vi "stop.vi"(8 "error in (no error)":errorcluster, 9 "CameraSettings":refnum<class "CamaraSettings.lvclass">, 10 "stop":bool, 11 "ProEM_WinX32 in":refnum<class "ProEM_WinX32.lvclass">) -> (0 "error out":errorcluster, 1 "imageSaved":bool, 2 "stopped?":bool, 3 "ProEM_WinX32 out":refnum<class "ProEM_WinX32.lvclass">)   [LabVIEW 2009, in "Hardware.lvlib" / "Channels.lvlib" / "ProEM_WinX32.lvclass"]
uses:
  ProEM_WinX32.lvclass
  Tools/CameraSettings/CamaraSettings.lvclass
  ProEM_WinX32.lvclass/ProEM_WinX32.ctl
  Camera/Camera.lvclass
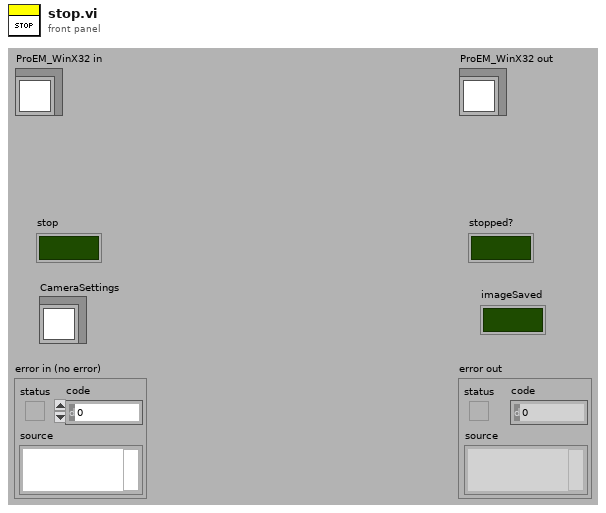
[diagram p1: front panel]
types:
  T1 = typedef "WINX32 Object Reference.ctl" = refnum<k1>
  T2 = typedef "WINX32 Data Members.ctl" = cluster{"WINX32Lib.IExpSetup":refnum<k7>, "WINX32Lib.IDocFile":refnum<k7>, "Result Image":T3, "Image to save":T3, "hardware present":bool, "started?":bool, "Image array from WINX":u16[][][], "raw images":cluster{"2D Image Array":u16[][]}[], "Camera active":bool, "images":T4, "Camera":T5}
  T3 = typedef "IMAQ Image.ctl" = refnum<image>
  T4 = typedef "WINX32 Image.ctl" = cluster{"processed":cluster{"Image":T3, u32}, "object":cluster{"Image":T3, u32}, "background":cluster{"Image":T3, u32}, "reference":cluster{"Image":T3, u32}, "mask":cluster{"Image":T3, u32}, "ROI Descriptor":cluster{"Global Rectangle":i32[], "Contours":cluster{"ID":enum32{"External", "Internal"}, "Type":enum32{"No Selection", "Point", "Line", "Rectangle", "Oval", "Polygon", "Free", "Unused1", "Unused2", "Unused3", "Broken Line", "Free Hand Line"}, "Coordinates":i32[]}[]}}
  T5 = typedef "Analyse - Camera.ctl" = cluster{"Bit Range(1023)":u32, "step(1.88)":dbl}
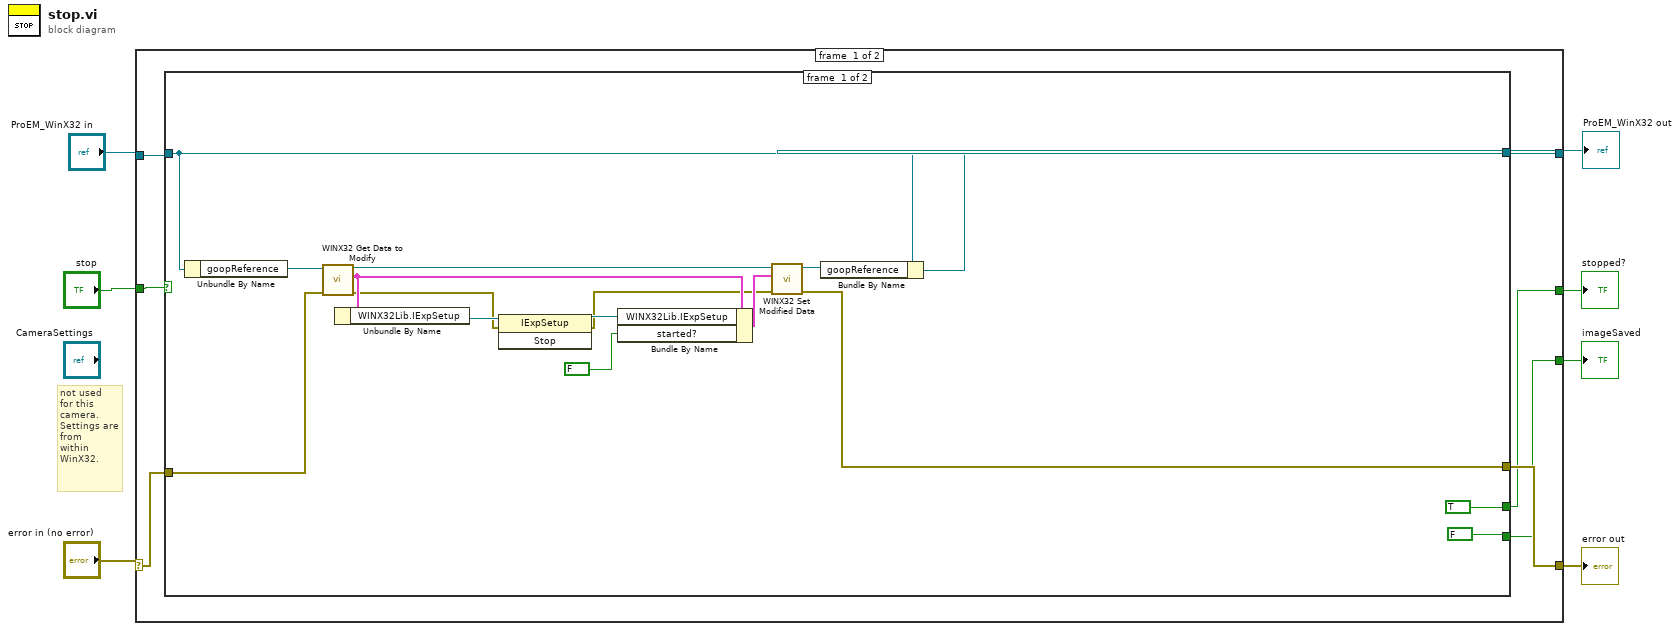
[diagram p0: block diagram]
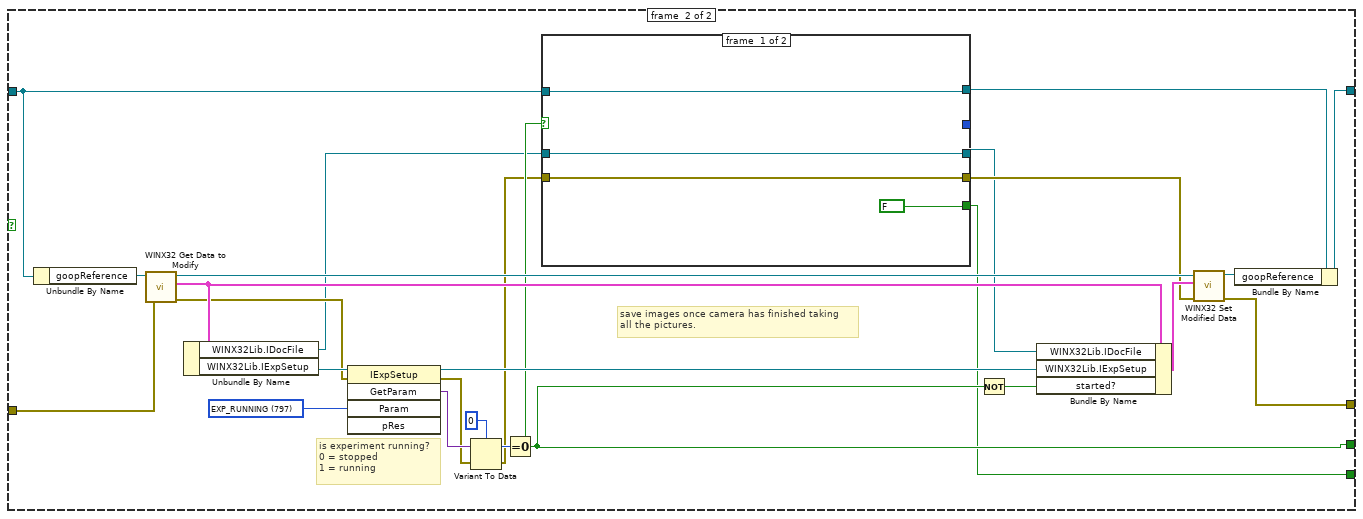
[diagram p2: hidden frame]
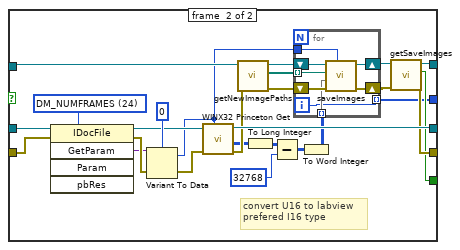
[diagram p3: hidden frame]
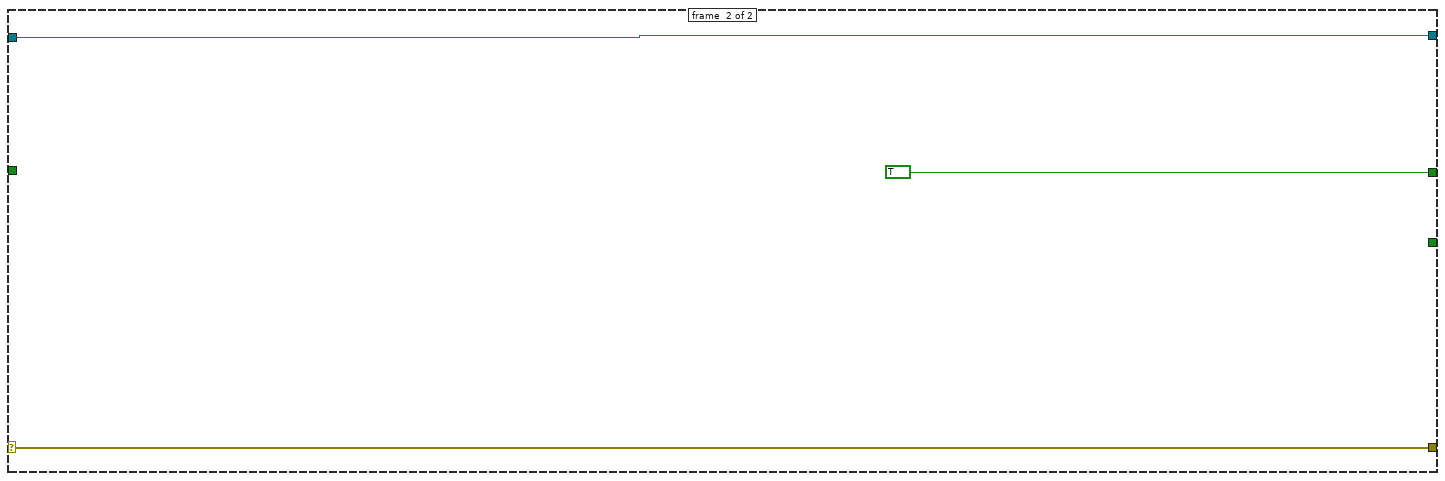
[diagram p4: hidden frame]
diagram:
  # "not used \nfor this\ncamera.\nSettings are\nfrom \nwithin \nWinX32."
  n1 = case shown="No Error" "error in (no error)" {
    selector: "error in (no error)" -> [w14 w95]
    tunnel: [w11 w96] -> w6
    tunnel: "ProEM_WinX32 in" -> [w12 w96]
    tunnel: [w10 w95] -> w4
    tunnel: "stop" -> [w13 _]
    tunnel: [w9 TRUE] -> w2
    tunnel: [w8 _] -> w1
    frame #0 {
      n2 = case shown="False" w13 {
        tunnel: w12 -> [w30 w32]
        tunnel: w14 -> [w27 w53]
        tunnel: [w29 w55] -> w11
        tunnel: [w17 w46] -> w10
        tunnel: [TRUE w38] -> w9
        tunnel: [FALSE w31] -> w8
        frame #0 {
          n3 = Unbundle By Name(w30) -> ("goopReference"=w28:T1)
          n4 = call <instrlib>:"WINX32 Get Data to Modify.vi"("error in (no error)"=w27, "reference"=w28) -> ("error out"=w23:errorcluster, "data"=w25:T2, "duplicate reference"=w21:T1)  [unwired: 2 in, 1 out]
          n5 = Unbundle By Name(w25) -> ("WINX32Lib.IExpSetup"=w26:refnum<k7>)
          n6 = invoke class="IExpSetup" method="Stop"(reference=w26, error in=w23) -> (reference out=w24:refnum<k7>, error out=w19:errorcluster)  [unwired: 1 in, 1 out]
          n7 = Bundle By Name(cluster=w25, "WINX32Lib.IExpSetup"=w24, "started?"=FALSE) -> (w20:T2)
          n8 = call <instrlib>:"WINX32 Set Modified Data.vi"("error in (no error)"=w19, "data"=w20, "reference"=w21) -> ("error out"=w17:errorcluster, "duplicate reference"=w22:T1)  [unwired: 3 in]
          n9 = Bundle By Name(cluster=w30, "goopReference"=w22) -> (w29:refnum<class "ProEM_WinX32.lvclass">)
        }
        frame #1 {
          w45 = 797 items=["EXP_ETACTUAL"=1, "EXP_SEQUENTS"=2, "EXP_ERROR"=3, "EXP_GETCAPS"=4, "EXP_GETPLSR"=5, "EXP_DETECTOR_BIT"=16, "EXP_RUNNING_APP"=23, "EXP_VIDEO_TYPE"=24, "EXP_CUSTOM_VIDEO_X"=25, "EXP_CUSTOM_VIDEO_Y"=26, "EXP_CUSTOM_VIDEO_FSTWIDTH"=27, "EXP_CUSTOM_VIDEO_LSTWIDTH"=28, "EXP_VIDEO_XDIM"=29, "EXP_VIDEO_YDIM"=30, "EXP_VIDEO_MAX_ZOOM"=31, "EXP_VIDEO_HORZ_PAN"=32, "EXP_VIDEO_VERT_PAN"=33, "EXP_WORD_MULTIPLIER"=34, "EXP_TARGET_ID"=35, "EXP_ADAPTER_ID"=36, "EXP_NUMADAPTORS"=37, "EXP_FORCE_PP_INIT"=38, "EXP_NOP_ADC"=39, "EXP_ACTUAL_TEMP"=40, "EXP_FORCE_AUTOSTOP"=41, "EXP_DEFAULT_VTCLK"=42, "EXP_MIN_VTCLK"=43, "EXP_MAX_VTCLK"=44, "EXP_DEFAULT_HTCLK"=45, "EXP_MIN_HTCLK"=46, "EXP_MAX_HTCLK"=47, "EXP_TIMING_STYLE"=48, "EXP_HEADSELECT"=49, "EXP_HORZPHASE"=50, "EXP_VERTPHASE"=51, "EXP_SPECIAL_SPEED"=52, "EXP_PRE_STRIPS"=53, "EXP_POST_STRIPS"=54, "EXP_PRE_LINES"=55, "EXP_POST_LINES"=56, "EXP_ACTIVE_LINES"=57, "EXP_ACTIVE_STRIPS"=58, "EXP_XFER_EXTRA"=59, "EXP_MIN_BLOCK"=60, "EXP_NUM_MIN_BLOCK"=61, "EXP_LOGIC_OUTPUT"=66, "EXP_VIDEO_BLANK"=67, "EXP_ZOOM_MODE_VIDEO"=68, "EXP_LEVEL_SYNC"=69, "EXP_DISABLE_LASER"=70, "EXP_ACQBACK_SHUTTER"=71, "EXP_ACQFLAT_SHUTTER"=72, "EXP_SMALL_CCD_MINEXP"=73, "EXP_LARGE_CCD_MINEXP"=74, "EXP_GATING_MODE"=75, "EXP_ILME_B1X"=76, "EXP_ILME_B2X"=77, "EXP_ILME_D1X"=78, "EXP_ILME_D2X"=79, "EXP_ILME_D4X"=80, "EXP_INIT_HW_ACCUM"=81, "EXP_5X_GAIN_ENABLE"=82, "EXP_RET_SRCCMP"=83, "EXP_EVENT_HANDLE"=84, "EXP_READOUT_MODE"=85, "EXP_SHUTTER_TYPE"=86, "EXP_USER_DEFINED_CHIP"=87, "EXP_USER_DEFINED_TIMING"=88, "EXP_CONTROLLER_VERSION"=89, "EXP_GET_CONTROLLER_VER"=90, "EXP_TTL_LINES"=91, "EXP_BIT_ADJUST"=92, "EXP_RESOLUTION"=93, "EXP_GAIN"=94, "EXP_ADC_RATE"=95, "EXP_ADC_TYPE"=96, "EXP_NUMBER_OF_CLEANS"=97, "EXP_NUM_OF_STRIPS_PER_CLN"=98, "EXP_INTERFACE_CARD"=99, "EXP_INTERRUPT"=100, "EXP_IO_ADDRESS1"=101, "EXP_IO_ADDRESS2"=102, "EXP_IO_ADDRESS3"=103, "EXP_HW_ROI"=104, "EXP_HW_BINNING"=105, "EXP_EDGE_TRIGGER"=106, "EXP_SHUTTER_CONTROL"=107, "EXP_RS170"=108, "EXP_RS170_COMPLEX"=109, "EXP_HW_RS170_LUT"=110, "EXP_RS170_INTENSITY_SCALING"=111, "EXP_RS170_OFFSET"=112, "EXP_RS170_PAN"=113, "EXP_RS170_ZOOM2X"=114, "EXP_RS170_ZOOM4X"=115, "EXP_RS170_BINNING"=116, "EXP_RS170_DECIMATION"=117, "EXP_HW_ACCUM"=118, "EXP_SHT_PREOPEN"=119, "EXP_STORE_STROBE"=120, "EXP_CONT_CLNS"=121, "EXP_TIMING_MODE"=122, "EXP_EXT_TRIGGER"=123, "EXP_EVENT_COUNTER"=124, "EXP_SW_TRIGGER"=125, "EXP_KINETICS_WINDOWSIZE"=126, "EXP_EXPOSURE"=127, "EXP_CONTROLLER_NAME"=128, "EXP_CCD_CHIP_NAME"=129, "EXP_BSWBINNING"=297, "EXP_EDGEENHANCE"=130, "EXP_BOXVIDEOGAIN"=131, "EXP_HSHADING_VALUE"=132, "EXP_VSHADING_VALUE"=133, "EXP_EDGEENHANCE_FLAG"=134, "EXP_SHADING_FLAG"=135, "EXP_GRAYSCALE"=136, "EXP_OFFSET"=137, "EXP_CCDGAIN"=138, "EXP_TEMPERATURE"=139, "EXP_MCPVOLTAGE"=140, "EXP_BOXEXPOSURE"=141, "EXP_ABC_FLAG"=142, "EXP_GAMMA_FLAG"=143, "EXP_AUTOBLACK_FLAG"=144, "EXP_AGC_FLAG"=145, "EXP_ODD_FIELD"=146, "EXP_FIELD_SELECT"=147, "EXP_RESET"=148, "EXP_EXTERN_ENABLE"=149, "EXP_CONTROLLERS_SUPPORTED"=150, "EXP_VTCLK"=151, "EXP_HTCLK"=152, "EXP_GATE_VS_CW"=153, "EXP_COM_PORT"=154, "EXP_US_UNITS"=156, "EXP_MS_UNITS"=157, "EXP_SEC_UNITS"=158, "EXP_MIN_UNITS"=159, "EXP_HRS_UNITS"=160, "EXP_FRAME_UNITS"=161, "EXP_SYNC_ASYNC"=162, "EXP_FOCUS_NFRAME"=163, "EXP_TIMEOUT"=164, "EXP_TIMEOUT_DEFAULT"=165, "EXP_HW_AUTOSTOP"=166, "EXP_RS170_INTEN_OFFSET"=167, "EXP_CONTROLLER_ALIVE"=168, "EXP_FOCUS_TYPE"=169, "EXP_FOCUS_ZOOM"=170, "EXP_FOCUS_PAN"=171, "EXP_MULTI_TAP_ROI"=172, "EXP_USE_INTERUPTS"=173, "EXP_DATA_ACQ_STATE"=174, "EXP_VERIFY_GOOD_VALUES"=175, "EXP_WHITE_CLAMP"=176, "EXP_BLACK_CLAMP"=177, "EXP_DELAY_TIME"=178, "EXP_READOUT_TIME"=179, "EXP_SW_DIAG"=180, "EXP_DIAG1"=181, "EXP_DIAG2"=182, "EXP_DIAG3"=183, "EXP_DIAG4"=184, "EXP_DIAG5"=185, "EXP_AorB_GROUP"=186, "EXP_ABSORBANCE_FLAG"=187, "EXP_ABSORBANCE_METHOD"=188, "EXP_ABSORBANCE_STRIPNUM"=189, "EXP_DMASIZE_VIA_DRIVER"=190, "EXP_DRIVERVERSION"=191, "EXP_NUM_DEVICES"=192, "EXP_ECPDMA_CHANNEL"=193, "EXP_CUSTOM_SHUTTER"=194, "EXP_ADC_OFFSET"=195, "EXP_CURRENT_READOUT_MODE"=196, "EXP_BANK_ADD"=197, "EXP_LUT_BANK"=198, "EXP_SETUP_STATUS"=201, "EXP_XY_GROUPING"=239, "EXP_MESSAGES_FLAG"=240, "EXP_TTL_LINE_TO_WAIT"=253, "EXP_DATA_COLLECTION_MODE"=258, "EXP_DATA_COLLECTION_TYPE"=262, "EXP_SKIPFRAMES"=274, "EXP_CLR_INT_CNTR"=276, "EXP_ENABLE_INT_CNTR"=277, "EXP_INT_CNTR"=278, "EXP_INTERNAL_SYNC_SRC"=279, "EXP_SW_EXTSYNC"=280, "EXP_PTG_PRESENT"=281, "EXP_ELEC_SHT"=282, "EXP_BOARDS_WITH_NVRAM"=283, "EXP_ANLGMASTER_ST143"=284, "EXP_ANLGSLAVE_ST143"=285, "EXP_DISPLAY_ST143"=286, "EXP_INTRFACE_ST143"=287, "EXP_SCANCONTROL_ST143"=288, "EXP_NUMBERFRAMES_IRQ"=204, "EXP_COOL_TYPE"=214, "EXP_HD_TYPE"=215, "EXP_INTENSIFER_GAIN"=216, "EXP_SHT_GATE_MODE"=217, "EXP_HD_CHECK"=218, "EXP_AMP_MODE"=219, "EXP_AMP_DIALOG"=247, "EXP_ANALOG_GAIN"=220, "EXP_HW_FIXES"=221, "EXP_PCI_CARDS"=222, "EXP_NOT_REVERSE"=223, "EXP_LOAD_NVRAM_DEFAULTS"=234, "EXP_CNTR_BRD"=235, "EXP_XDIMHW"=237, "EXP_YDIMHW"=238, "EXP_SPECIAL_FAST_RDOUT"=254, "EXP_SPCL_FAST_Y_DIM"=255, "EXP_SPCL_FAST_X_DIM"=256, "EXP_SPCL_FAST_Y_INDEX"=257, "EXP_SHUTTER_COMP_TIME_MS"=266, "EXP_NVRAM_AVAIL"=267, "EXP_NUMBER_AGAIN_AVAIL"=269, "EXP_SENSOR_TYPE"=270, "EXP_EVENT_TYPE"=292, "EXP_ANTI_BLOOMING"=293, "EXP_FAST_PULSE_ENABLE"=233, "EXP_USE_HEADCALIB"=296, "EXP_TEMP_STATUS"=301, "EXP_MULTIPLE_READMODES_LIVE"=302, "EXP_FIRST_ACQUIRE_FLAG"=303, "EXP_ANTI_BLOOMING_CONTROL"=304, "EXP_PRE_HORZ_DELAY"=305, "EXP_NVRAM_TRIES"=306, "EXP_XASCEND"=307, "EXP_YASCEND"=308, "EXP_ALT_TIMING"=309, "EXP_SHUTTER_PRE_COMP"=310, "EXP_PVCAM_POSSIBLE"=311, "EXP_ADC_IN_NVRAM"=312, "EXP_PASSTHRU_MODE"=313, "EXP_FIRMWAREVERSION"=314, "EXP_IMMEDIATE_SHUTTER"=315, "EXP_STAGE2_TEMP"=316, "EXP_AVGAIN_ENABLED"=317, "EXP_AVGAIN_SETPOINT"=318, "EXP_AVGAIN"=319, "EXP_AVGAIN_CALIB_TEMP"=320, "EXP_AVGAIN_CALIB_COEFF1"=321, "EXP_AVGAIN_CALIB_COEFF2"=322, "EXP_AVGAIN_CALIB_COEFF3"=323, "EXP_AVGAIN_CALIB_COEFF4"=324, "EXP_AVGAIN_CALIB_COEFF5"=325, "EXP_FORCE_READOUT_MODE"=326, "EXP_RESET_DATACOLLECTION"=327, "EXP_ACTIVE_SUBFRAME"=328, "EXP_PV_READOUT_PORT"=514, "EXP_CLASSNAME"=775, "EXP_FLATFLDNAME"=776, "EXP_DARKNAME"=777, "EXP_SETUPNAME"=778, "EXP_ACCESSNAME"=779, "EXP_DATFILENAME"=780, "EXP_ABSORBFILENAME"=781, "EXP_BLEMISHFILENAME"=782, "EXP_COSMICFILENAME"=783, "EXP_FILEINCBASENAME"=784, "EXP_YTNAME"=785, "EXP_DEVNAME"=786, "EXP_USEROI"=787, "EXP_DOBLEMISH"=788, "EXP_DOABSORB"=789, "EXP_DOCOSMIC"=790, "EXP_COSMICSENS"=791, "EXP_ABSORBSTRIP"=792, "EXP_DATATYPE"=793, "EXP_OVERWRITECONFIRM"=794, "EXP_FILEINCENABLE"=795, "EXP_FILEINCCOUNT"=796, "EXP_RUNNING"=797, "EXP_SAVEROPT"=798, "EXP_TIME_UNITS"=799, "EXP_FILEACCESS"=800, "EXP_AUTOSAVE"=801, "EXP_NEWWINDOW"=802, "EXP_XDIM"=803, "EXP_YDIM"=804, "EXP_XDIMDET"=805, "EXP_YDIMDET"=806, "EXP_ROIMODE"=807, "EXP_NUMREPEATSEXP"=808, "EXP_NUMACCUMSEXP"=809, "EXP_THREADSTATE"=810, "EXP_USEMINTHRESHOLDING"=811, "EXP_MINTHRESHOLDVALUE"=812, "EXP_USEMAXTHRESHOLDING"=813, "EXP_MAXTHRESHOLDVALUE"=814, "EXP_RUNNING_EXPERIMENT"=815, "EXP_THRESHOLD_DEMAND_UPDATE"=816, "EXP_ROICOUNT"=817, "EXP_ACCUMS"=818, "EXP_CACCUMS"=819, "EXP_CSEQUENTS"=820, "EXP_PHOTON_ESTIMATION_ENABLE"=821, "EXP_PHOTON_MAXTIME"=822, "EXP_PHOTON_MAXTIMEUNIT"=823, "EXP_CUSTOMFILTER_ENABLE"=824, "EXP_CUSTOMFILTER_SIZE"=825, "EXP_LOOKUPTABLE_ENABLE"=826, "EXP_BSHOWWINDOW"=827, "EXP_BBACKSUBTRACT"=828, "EXP_BDOFLATFIELD"=829, "EXP_ASCIIOUTPUTFILE"=830, "EXP_ASCIIOUTPUT_DELIMITER"=831, "EXP_ASCIIOUTPUT_TERMINATOR"=832, "EXP_FFTYPE"=833, "EXP_BGTYPE"=834, "EXP_COSGRASS"=835, "EXP_RUNASCONFIRM"=836, "EXP_RUNASRUNACCESS"=837, "EXP_DATAFILETYPE"=838, "EXP_ROTATE"=839, "EXP_FLIP"=840, "EXP_REVERSE"=841, "EXP_SWBINNING"=842, "EXP_AUTOSTORE"=843, "EXP_XBINNED"=844, "EXP_YBINNED"=845, "EXP_NUMPATTERNS"=846, "EXP_EXPERIMENTTIME"=847, "EXP_ASYNCSEQUENTIALS"=848, "EXP_SEQUENTIALS"=849, "EXP_CSEQUENTIALS"=850, "EXP_AUTOD"=851, "EXP_EXPOSURETIME"=852, "EXP_EXPOSURETIME_UNITS"=853, "EXP_ACQMODE"=854, "EXP_DMASIZE_PVCAM"=855, "EXP_INITIALIZE"=856, "EXP_CELL_X_SIZE"=857, "EXP_CELL_Y_SIZE"=858, "EXP_X_GAP_SIZE"=859, "EXP_Y_GAP_SIZE"=860] ("Param")
          # "is experiment running?\n0 = stopped\n1 = running"
          # "save images once camera has finished taking\nall the pictures."
          n10 = Unbundle By Name(w32) -> ("goopReference"=w54:T1)
          n11 = call <instrlib>:"WINX32 Get Data to Modify.vi"("error in (no error)"=w53, "reference"=w54) -> ("error out"=w50:errorcluster, "data"=w51:T2, "duplicate reference"=w48:T1)  [unwired: 2 in, 1 out]
          n12 = Unbundle By Name(w51) -> ("WINX32Lib.IDocFile"=w35:refnum<k7>, "WINX32Lib.IExpSetup"=w52:refnum<k7>)
          n13 = invoke class="IExpSetup" method="GetParam"(reference=w52, error in=w50, "Param"=w45) -> (reference out=w39:refnum<k7>, error out=w42:errorcluster, "GetParam"=w44:variant)  [unwired: 2 in, 2 out]
          n14 = Variant To Data(error in=w42, Variant=w44, type=u16 0) -> (error out=w37:errorcluster, data=w41:u16)
          n15 = Equal To 0?(x=w41) -> (x = 0?=w38:bool)
          n16 = case shown="True" w38 {
            tunnel: w35 -> [w59 w85]
            tunnel: w37 -> [w58 w83]
            tunnel: [w58 w62] -> w36
            tunnel: [w59 w78] -> w34
            tunnel: [w57 w64] -> w33
            tunnel: w32 -> [w57 w76]
            tunnel: [FALSE w61] -> w31
            tunnel: [_ w60] -> _
            frame #0 {
            }
            frame #1 {
              w84 = 24 items=["DM_XDIMDET"=1, "DM_YDIMDET"=2, "DM_TIMINGMODE"=3, "DM_EXPOSEC"=4, "DM_DETTYPE"=5, "DM_XDIM"=6, "DM_YDIM"=7, "DM_ASYNEN"=8, "DM_DATATYPE"=9, "DM_PIXELSIZE"=10, "DM_MINBLK"=11, "DM_NUMMINBLK"=12, "DM_ADCRATE"=13, "DM_ADCTYPE"=14, "DM_ADCRESOLUTION"=15, "DM_ADCBITADJUST"=16, "DM_GAIN"=17, "DM_GEOMETRIC"=18, "DM_CLEANS"=19, "DM_NUMSKPPERCLN"=20, "DM_FILEVERSION"=21, "DM_SWVERSION"=22, "DM_CONTROLLERTYPE"=23, "DM_NUMFRAMES"=24, "DM_MAXINTENSITY"=25, "DM_MININTENSITY"=26, "DM_SHUTTERTYPE"=27, "DM_SHUTTERCOMP"=28, "DM_READOUTMODE"=29, "DM_WINDOWSIZE"=30, "DM_CLKSPD"=31, "DM_KINTRIGMODE"=32, "DM_CLKSPD_us"=33, "DM_INTERFACETYPE"=34, "DM_NOT_IN_USE_0"=35, "DM_NOT_IN_USE_1"=36, "DM_NOT_IN_USE_2"=37, "DM_NOT_IN_USE_3"=38, "DM_NOT_IN_USE_4"=39, "DM_NOT_IN_USE_5"=40, "DM_COSMICAPPLIED"=41, "DM_COSMICTYPE"=42, "DM_COSMICTHRESHOLD"=43, "DM_BLEMISHAPPLIED"=44, "DM_FLATFIELDAPPLIED"=45, "DM_BACKGROUNDAPPLIED"=46, "DM_ACCUMS"=47, "DM_HWACCUMS"=48, "DM_NOT_IN_USE_6"=49, "DM_NOT_IN_USE_7"=50, "DM_NOT_IN_USE_8"=51, "DM_STORESYNC"=52, "DM_SWMADE"=53, "DM_FLATFIELDNAME"=54, "DM_BACKSUBNAME"=55, "DM_XLABEL"=56, "DM_YLABEL"=57, "DM_DLABEL"=58, "DM_FILEDATE"=59, "DM_BLEMISHFILE"=60, "DM_USERINFO"=61, "DM_USERCOMMENT1"=62, "DM_USERCOMMENT2"=63, "DM_USERCOMMENT3"=64, "DM_USERCOMMENT4"=65, "DM_USERCOMMENT5"=66, "DM_xCAL_OFFSET"=67, "DM_xCAL_FACTOR"=68, "DM_xCAL_CURR_UNIT"=69, "DM_xCAL_STRING"=70, "DM_xCAL_VALID"=71, "DM_xCAL_INPUT_UNIT"=72, "DM_xCAL_POLYNOM_UNIT"=73, "DM_xCAL_CALIB_COUNT"=74, "DM_xCAL_PXL_POS"=75, "DM_xCAL_PXL_VAL"=76, "DM_xCAL_POLYNOM_ORDER"=77, "DM_xCAL_COEFFS"=78, "DM_xCAL_LASERLINE"=79, "DM_xCAL_FILE_LABEL"=80, "DM_NUMROI"=81, "DM_ROI_STARTX"=82, "DM_ROI_ENDX"=83, "DM_ROI_GP_X"=84, "DM_ROI_STARTY"=85, "DM_ROI_ENDY"=86, "DM_ROI_GP_Y"=87, "DM_CONTROLLERNUM"=88, "DM_DEFAULTTYPE"=89, "DM_FRAMECOUNT"=90, "DM_LASTFRAMERDY"=91, "DM_FRAMEINPROS"=92, "DM_SCANCOUNT"=93, "DM_TEMPFLAG"=94, "DM_STOREFLAG"=95, "DM_FRAMESIZE"=96, "DM_ISDISPLAYED"=97, "DM_INUSE"=98, "DM_LASTVALUE"=99, "DM_STOREFLAGSAVE"=100, "DM_YTFLAG"=101, "DM_YT_AREAS_EQUS"=102, "DM_YT_POINTS_TAKEN"=103, "DM_FILENAME"=104, "DM_FILETITLE"=105, "DM_DOCTYPE"=106, "DM_NUMEXPREPEATS"=107, "DM_NUMEXPACCUMS"=108, "DM_UPDATEVIEWS"=109, "DM_PULSEFILENAME"=110, "DM_PULSEREPWIDTH"=111, "DM_PULSEREPDELAY"=112, "DM_CONTROLLERVERSION"=113, "DM_LOGICOUTPUT"=114, "DM_VIRTUALCHIPFLAG"=115, "DM_PULSERTYPE"=116, "DM_AMPHICAPLOWNOISE"=117, "DM_VCHIPXDIM"=118, "DM_VCHIPYDIM"=119, "DM_PIMAXUSED"=120, "DM_PIMAXMODE"=121, "DM_SHUTTERCONTROL"=122, "DM_ABSORBLIVE"=123, "DM_ABSORBMODE"=124, "DM_ABSORBSTRIPNUM"=125, "DM_THRESHOLDMINLIVE"=126, "DM_THRESHOLDMAXLIVE"=127, "DM_SPECAUTOSPECTROMODE"=128, "DM_SPECGLUEFLAG"=129, "DM_PULSERMODE"=130, "DM_PULSERONCHIPACCUMS"=131, "DM_PULSERREPEATEXP"=132, "DM_PULSESEQINCMODE"=133, "DM_ADCOFFSET"=134, "DM_ABSORBFILENAME"=135, "DM_NUMROISINEXPERIMENT"=136, "DM_SPECMIRRORLOCATION"=137, "DM_SPECSLITLOCATION"=138, "DM_SPECMIRRORPOS"=139, "DM_READOUTTIME"=140, "DM_DETTEMPERATURE"=141, "DM_DELAYTIME"=142, "DM_THRESHOLDMINVAL"=143, "DM_THRESHOLDMAXVAL"=144, "DM_SPECCENTERWLNM"=145, "DM_SPECGLUESTARTWLNM"=146, "DM_SPECGLUEENDWLNM"=147, "DM_SPECGLUEMINOVRLPNM"=148, "DM_SPECGLUEFINALRESNM"=149, "DM_PULSESEQSTARTWIDTH"=150, "DM_PULSESEQENDWIDTH"=151, "DM_PULSESEQSTARTDELAY"=152, "DM_PULSESEQENDDELAY"=153, "DM_SPECSLITPOS"=154, "DM_AUTOCLEANSACTIVE"=155, "DM_USECONTCLEANSINST"=156, "DM_CUSTOMCHIPFLAG"=157, "DM_XPREPIXELS"=158, "DM_XPOSTPIXELS"=159, "DM_YPREPIXELS"=160, "DM_YPOSTPIXELS"=161, "DM_CUSTOMTIMINGFLAG"=162, "DM_CANDOVIRTUALCHIPFLAG"=163, "DM_PIMAXGAIN"=164, "DM_PIMAX2NSBRDUSED"=165, "DM_TRIGGEREDMODEFLAG"=166, "DM_CONTINUOUSCLEANSFLAG"=167, "DM_EXTERNALTRIGGERFLAG"=168, "DM_EXPERIMENTTIMELOCAL"=169, "DM_EXPERIMENTTIMEUTC"=170, "DM_EXPOSUNITS"=171, "DM_SPECSLITPOSUNITS"=172, "DM_SPECGROOVES"=173, "DM_AVGAINUSED"=174, "DM_AVGAIN"=175, "DM_ANALOGGAIN"=176, "DM_SPECTYPE"=177, "DM_SPECMODEL"=178, "DM_PULSEBURSTUSED"=179, "DM_PULSEBURSTCOUNT"=180, "DM_PULSEBURSTPERIOD"=181, "DM_PULSEBRACKETUSED"=182, "DM_PULSEBRACKETTYPE"=183, "DM_PULSETIMECONSTFAST"=184, "DM_PULSEAMPLITUDEFAST"=185, "DM_PULSETIMECONSTSLOW"=186, "DM_PULSEAMPLITUDESLOW"=187] ("Param")
              # "convert U16 to labview \nprefered I16 type"
              n17 = invoke class="IDocFile" method="GetParam"(reference=w85, error in=w83, "Param"=w84) -> (reference out=w77:refnum<k7>, error out=w82:errorcluster, "GetParam"=w81:variant)  [unwired: 2 in, 2 out]
              n18 = Variant To Data(error in=w82, Variant=w81, type=u16 0 ("number of images")) -> (error out=w80:errorcluster, data=w71:u16)
              n19 = call <instrlib>:"WINX32 Princeton Get.vi"("number of images"=w71, "error in"=w80, "WINX32Lib.IDocFile"=w77) -> ("error out"=w74:errorcluster, "Image array"=w67:u16[][][], "WINX32Lib.IDocFile copy"=w78:refnum<k7>)  [unwired: 4 in]
              n20 = call "getNewImagePaths.vi"("error in (no error)"=w74, "Camera in"=w76) -> ("error out"=w73:errorcluster, "ImagePaths"=w72:path[], "Camera out"=w75:refnum<class "ProEM_WinX32.lvclass">)  [unwired: 7 in]
              n21 = To Long Integer(number=w67) -> (32bit integer=w69:i32[][][])
              n22 = Subtract(x=w69, y=32768) -> (x-y=w70:i32[][][])
              n23 = To Word Integer(number=w70) -> (16bit integer=w66:i16[][][])
              n24 = for {
                shift-right: [w90] -> w65
                shift-left: w75 -> [w92]
                shift-right: [w93] -> w63
                shift-left: w73 -> [w91]
                tunnel: w72 -> [w89] mode=indexing
                tunnel: w66 -> [w88] mode=indexing
                tunnel: w71 -> [w87]
                tunnel: [w86] -> w60 mode=indexing
                i -> [w86]
                n25 = call "saveImages.vi"("totalImageNumber"=w87, "error in (no error)"=w91, "I16bit image data"=w88, "Path"=w89, "ProEM_WinX32 in"=w92) -> ("error out"=w93:errorcluster, "ProEM_WinX32 out"=w90:refnum<class "ProEM_WinX32.lvclass">)  [unwired: 5 in]
              }
              n26 = call "getSaveImages.vi"("error in (no error)"=w63, "Camera in"=w65) -> ("error out"=w62:errorcluster, "saveImages?"=w61:bool, "Camera out"=w64:refnum<class "ProEM_WinX32.lvclass">)  [unwired: 7 in]
            }
          }
          n27 = Not(x=w38) -> (.not. x?=w40:bool)
          n28 = Bundle By Name(cluster=w51, "WINX32Lib.IDocFile"=w34, "WINX32Lib.IExpSetup"=w39, "started?"=w40) -> (w47:T2)
          n29 = call <instrlib>:"WINX32 Set Modified Data.vi"("error in (no error)"=w36, "data"=w47, "reference"=w48) -> ("error out"=w46:errorcluster, "duplicate reference"=w49:T1)  [unwired: 3 in]
          n30 = Bundle By Name(cluster=w33, "goopReference"=w49) -> (w55:refnum<class "ProEM_WinX32.lvclass">)
        }
      }
    }
    frame #1 {
    }
  }
  "error out" <- w4
  "ProEM_WinX32 out" <- w6
  "imageSaved" <- w1
  "stopped?" <- w2
